vi "SetupM1M3Events.vi"(8 "error in (no error)":errorcluster, 11 "Model in":refnum<class "Model.lvclass">) -> (0 "error out":errorcluster, 3 "Model out":refnum<class "Model.lvclass">)   [LabVIEW 2016, in "Model.lvclass"]
uses:
  Model.lvclass
  M1M3 Support Events/M1M3 Support Events.lvclass
  Model.lvclass/Model.ctl
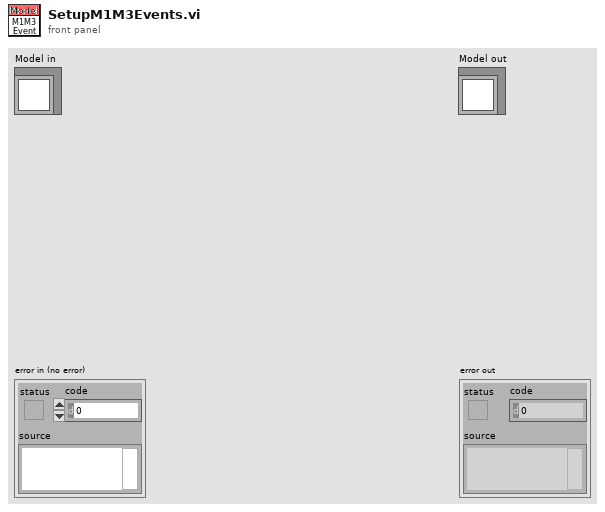
[diagram p1: front panel]
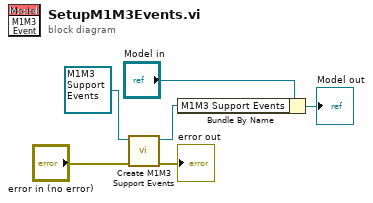
[diagram p0: block diagram]
diagram:
  n1 = call "Create M1M3 Support Events.vi"("error in (no error)"="error in (no error)", "M1M3 Support Events in"=refnum<class "M1M3 Support Events.lvclass"> refnum ("M1M3 Support Events.lvclass")) -> ("error out"=→"error out":errorcluster, "M1M3 Support Events out"=w2:refnum<class "M1M3 Support Events.lvclass">)  [unwired: 8 in]
  n2 = Bundle By Name(cluster="Model in", "M1M3 Support Events"=w2) -> (→"Model out":refnum<class "Model.lvclass">)
